vi "Database_Insert_Patient.vi"(11 "Patient_ID":string) -> (3 "Patient List":string[][](array[string]))   [LabVIEW 2013, in "Medimatic.lvlib"]
uses:
  Medimatic.lvlib
  Globals/DataPathGlobalVariable.vi
  <userlib>/LVT/SQLite/Core/Insert/SQLite_Insert Row.vi
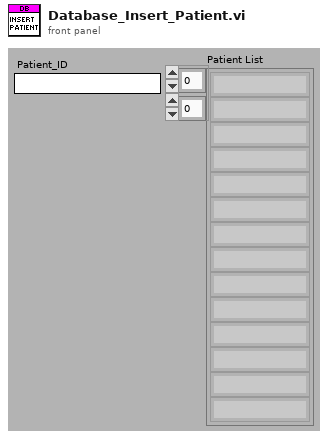
[diagram p1: front panel]
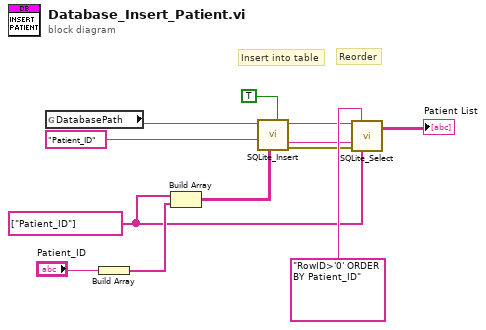
[diagram p0: block diagram]
diagram:
  w2 = string[] ["Patient_ID"]
  # "Reorder"
  # "Insert into table"
  n1 = global read "DataPathGlobalVariable.vi" "DatabasePath"() -> (w11:string)
  n2 = Build Array("Patient_ID") -> (w5:string[])
  n3 = Build Array(w2, w5) -> (w4:string[][])
  n4 = call-poly <userlib>:"SQLite_Insert.vi"("Transpose"=TRUE, "Column/Value Pairs"=w4, "Table Name"="Patient_ID", "DB Path"=w11) -> ("error out"=w7:errorcluster, "Tabe Name Out"=w6:string, "DB Path Out"=w8:string)  [unwired: 3 in]
  n5 = call <userlib>:"SQLite_Select.vi"("DB Path"=w8, "Where Clause"="RowID>'0' ORDER BY Patient_ID", "Table Name"=w6, "error in (no error)"=w7, "Columns"=w2) -> ("Results"=→"Patient List":string[][])  [unwired: 7 in, 3 out]
